vi "GetIMUData.vi"(8 "error in (no error)":errorcluster, 11 "Channel Name":tag="A/I2C") -> (0 "error out":errorcluster, 2 "GyroData":T1, 3 "AccelData":T1)   [LabVIEW 2019]
uses:
  MPU6050/DeviceAddresses.ctl
  <vilib>/myRIO/Instrument Drivers/Onboard IO/I2C/typedefs/I2C User Configuration.ctl
  <vilib>/myRIO/Instrument Drivers/Onboard IO/I2C/typedefs/I2C Transfer Rate.ctl
  LIFA MPU-60X0 LV9/AccelFullScaleRanges.ctl
  LIFA MPU-60X0 LV9/GyroFullScaleRanges.ctl
  <vilib>/myRIO/Instrument Drivers/Onboard IO/I2C/typedefs/I2C Reference.ctl
  <vilib>/myRIO/Common/Instrument Driver Framework/Utilities/typedefs/myRIO Generic Hardware Reference.ctl
  <vilib>/myRIO/Common/Instrument Driver Framework/Utilities/typedefs/Hardware Version Enum.ctl
  <vilib>/myRIO/Common/Instrument Driver Framework/Utilities/typedefs/myRIO v1.0 Reference.ctl
  <vilib>/myRIO/Common/Instrument Driver Framework/Utilities/typedefs/Generic FPGA Reference.ctl
  <vilib>/myRIO/Common/Instrument Driver Framework/myRIO v1.0/I2C/typedefs/I2C Channels Enum.ctl
  <vilib>/myRIO/Instrument Drivers/Onboard IO/I2C/typedefs/I2C Configuration.ctl
  <vilib>/userDefined/High Color/nirio_resource_hc.ctl
  <vilib>/myRIO/Common/Instrument Driver Framework/myRIO v1.0/I2C/vis/myRIO v1.1 Open I2C.vi
  <vilib>/myRIO/Common/Instrument Driver Framework/Utilities/vis/Validate Channels.vi
  <vilib>/myRIO/Common/Instrument Driver Framework/myRIO v1.0/I2C/vis/myRIO v1.0 Reserve I2C.vi
  <vilib>/myRIO/Common/Instrument Driver Framework/myRIO v1.0/I2C/vis/myRIO v1.0 Close I2C.vi
  <vilib>/myRIO/Common/Instrument Driver Framework/myRIO v1.0/I2C/vis/myRIO v1.0 Build MUX Configuration I2C.vi
  <vilib>/myRIO/Common/Instrument Driver Framework/myRIO v1.0/Resource Manager/vis/myRIO v1.0 Reserve Channel List.vi
  <vilib>/myRIO/Common/Instrument Driver Framework/myRIO v1.0/I2C/vis/myRIO v1.0 Unreserve I2C.vi
  <vilib>/myRIO/Common/Instrument Driver Framework/myRIO v1.0/Resource Manager/vis/myRIO v1.0 Create Configuration List.vi
  <vilib>/myRIO/Common/Instrument Driver Framework/myRIO v1.0/Resource Manager/vis/myRIO v1.0 Reserve Channel.vi
  <vilib>/myRIO/Common/Instrument Driver Framework/myRIO v1.0/Resource Manager/vis/myRIO v1.0 Unreserve Channel.vi
  <vilib>/myRIO/Common/Instrument Driver Framework/myRIO v1.0/Resource Manager/vis/myRIO v1.0 Unreserve Channel List.vi
  <vilib>/myRIO/Common/Instrument Driver Framework/myRIO v1.0/Resource Manager/vis/myRIO v1.0 Build Mutex Name.vi
  <vilib>/Utility/VariantDataType/GetNumericInfo.vi
  <vilib>/Utility/error.llb/Error Cluster From Error Code.vi
  <vilib>/myRIO/Common/Instrument Driver Framework/myRIO v1.0/myRIO v1.1 Open.vi
  <vilib>/myRIO/Common/Instrument Driver Framework/Utilities/vis/IO Manager.vi
  <vilib>/myRIO/Common/Instrument Driver Framework/Utilities/vis/Configuration Manager.vi
  <vilib>/myRIO/Common/Instrument Driver Framework/myRIO v1.0/Resource Manager/vis/myRIO v1.0 Configure IO.vi
  <vilib>/myRIO/Common/Instrument Driver Framework/myRIO v1.0/myRIO v1.0 Close.vi
  <vilib>/myRIO/Common/Instrument Driver Framework/myRIO v1.0/I2C/vis/myRIO v1.0 Configure I2C.vi
  <vilib>/myRIO/Common/Instrument Driver Framework/myRIO v1.0/I2C/vis/myRIO v1.0 Shutdown I2C.vi
  <vilib>/myRIO/Instrument Drivers/Onboard IO/I2C/vis/myRIO I2C Open.xnode
  <vilib>/myRIO/Instrument Drivers/Onboard IO/I2C/I2C.lvlib
  LIFA MPU-60X0 LV9/LIFA MPU-60X0.lvlib
panel:
  in  "Stop Button":bool=TRUE
  out "Temperature (°C)":dbl(slide) scale=0.0..100.0
  out "Gyro Data":T1(graph)
  out "Accelerometer Data":T1(graph)
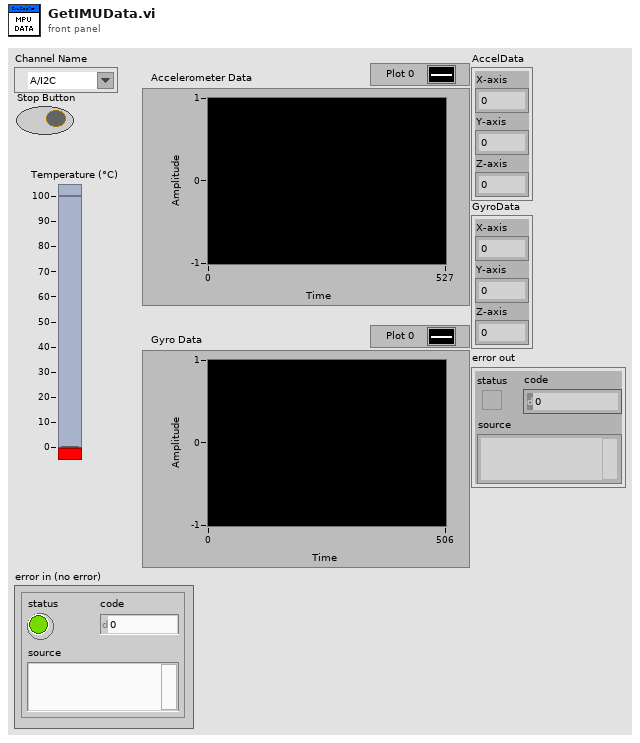
[diagram p1: front panel]
types:
  T1 = cluster{"X-axis":i16, "Y-axis":i16, "Z-axis":i16}
  T2 = typedef "LIFA MPU-60X0.lvlib/GyroFullScaleRanges.ctl" = enum8{"±250 °/s", "±500 °/s", "±1000 °/s", "±2000 °/s"}
  T3 = typedef "LIFA MPU-60X0.lvlib/AccelFullScaleRanges.ctl" = enum16{"±2g", "±4g", "±8g", "±16g"}
  T4 = typedef "I2C.lvlib/I2C User Configuration.ctl" = cluster{"I2C Transfer Rate":T5}
  T5 = typedef "I2C.lvlib/I2C Transfer Rate.ctl" = enum16{"Standard mode (100 kbps)", "Fast mode (400 kbps)"}
  T6 = typedef "DeviceAddresses.ctl" = u8
  T7 = typedef "I2C.lvlib/I2C Reference.ctl" = cluster{"myRIO Reference":T8, "I2C Channels Enum":T12, "I2C Configuration":T13}
  T8 = typedef "myRIO Generic Hardware Reference.ctl" = cluster{"myRIO Model":T9, "myRIO Hardware Reference":T10}
  T9 = typedef "Hardware Version Enum.ctl" = enum16{"Unknown", "myRIO-1900", "myRIO-1950", "roboRIO", "NI ELVIS RIO CM", "ELVIS III"}
  T10 = typedef "myRIO v1.0 Reference.ctl" = cluster{"Generic FPGA Reference":T11, "Allow multiple opens":bool}
  T11 = typedef "Generic FPGA Reference.ctl" = refnum<k20>
  T12 = typedef "I2C Channels Enum.ctl" = enum16{"Not Connected", "A/I2C", "B/I2C", "I2C/I2C"}
  T13 = typedef "I2C.lvlib/I2C Configuration.ctl" = cluster{"I2C Transfer Rate":T5}
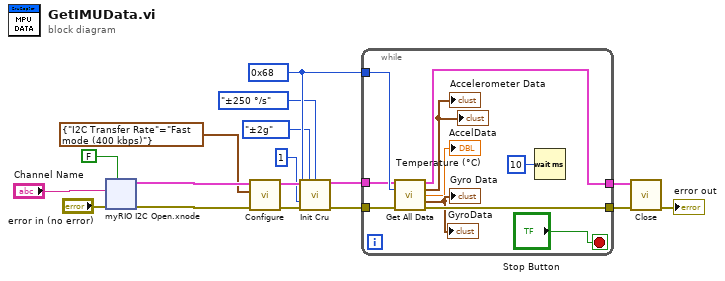
[diagram p0: block diagram]
diagram:
  w14 = T6 104 items=["0x68"=104, "0x69"=105] ("Device Address")
  n1 = xnode "myRIO I2C Open.xnode"("error in (no error)"="error in (no error)", "Allow multiple opens?"=FALSE, "Channel Name"="Channel Name") -> ("error out"=w9:errorcluster, "I2C Ref Out"=w11:T7)
  n2 = call <vilib>:"Configure.vi"("error in (no error)"=w9, "I2C User Configuration"=T4 {"I2C Transfer Rate"=enum."Fast mode (400 kbps)"}, "I2C Ref In"=w11) -> ("error out"=w8:errorcluster, "I2C Ref Out"=w10:T7)  [unwired: 7 in]
  n3 = call "Init Cru.vi"("I2C Ref In"=w10, "Accel Full Scale Range"=AccelFullScaleRanges."±2g", "Gyro Full Scale Range"=GyroFullScaleRanges."±250 °/s", "Device Address"=w14, "Clock Source"=u8 1, "error in (no error)"=w8) -> ("I2C Ref Out"=w12:T7, "error out"=w13:errorcluster)  [unwired: 8 in]
  n4 = while {
    tunnel: w13 -> [w27]
    tunnel: w14 -> [w26]
    tunnel: [w25] -> w16
    tunnel: [w24] -> w15
    tunnel: w12 -> [w19]
    stop <- "Stop Button" stop-if-true
    n5 = call "Get All Data.vi"("I2C Ref In"=w19, "Device Address"=w26, "error in (no error)"=w27) -> ("I2C Ref Out"=w25:T7, "Accel Data"=→"Accelerometer Data" →"AccelData":T1, "Temperature (°C)"=→"Temperature (°C)":dbl, "Gyro Data"=→"Gyro Data" →"GyroData":T1, "error out"=w24:errorcluster)  [unwired: 8 in]
    n6 = Wait (ms)(milliseconds to wait=u32 10) -> ()  [unwired: 1 out]
  }
  n7 = call <vilib>:"Close.vi"("error in (no error)"=w15, "I2C Ref In"=w16) -> ("error out"=→"error out":errorcluster)  [unwired: 9 in]
